vi "SendCmd.vi"(6 "HighPriority (F)":bool, 7 "UICmd":string, 8 "error in":errorcluster, 9 "Control Data":variant, 10 "Control Label":string, 11 "Queue in":refnum<queue>) -> (0 "error out":errorcluster)   [LabVIEW 2018, in "UI_Library.lvlib"]
uses:
  UI_Library.lvlib
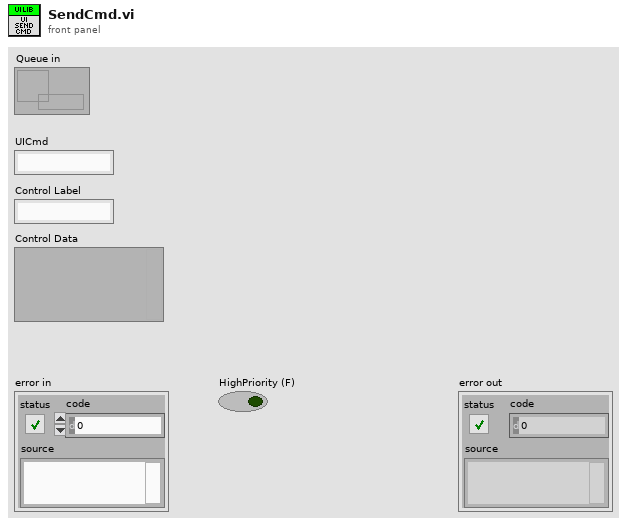
[diagram p1: front panel]
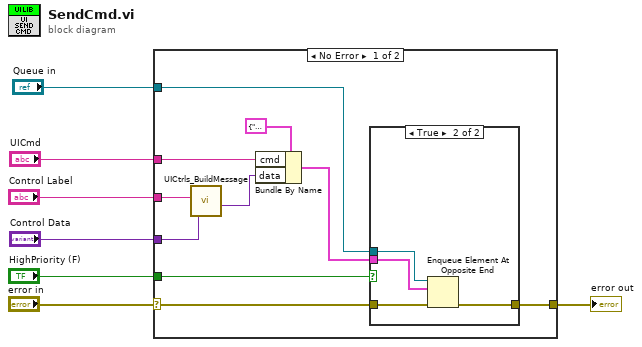
[diagram p0: block diagram]
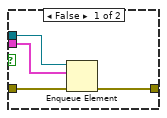
[diagram p2: hidden frame]
diagram:
  n1 = case shown="No Error" "error in" {
    selector: "error in" -> [w9 w26]
    tunnel: "Queue in" -> [w17 _]
    tunnel: "Control Label" -> [w13 _]
    tunnel: "Control Data" -> [w12 _]
    tunnel: "UICmd" -> [w11 _]
    tunnel: "HighPriority (F)" -> [w10 _]
    tunnel: [w8 w26] -> w7
    frame No Error {
      n2 = call "UICtrls_BuildMessage.vi"("Control Label"=w13, "Control Data"=w12) -> ("Data"=w14:variant)  [unwired: 6 in]
      n3 = Bundle By Name(cluster=cluster{"cmd":string, "data":variant} {"cmd"="", "data"=variant} ("element"), "cmd"=w11, "data"=w14) -> (w15:cluster{"cmd":string, "data":variant})
      n4 = case shown="True" w10 {
        tunnel: w17 -> [w21 w24]
        tunnel: w15 -> [w20 w23]
        tunnel: w9 -> [w19 w25]
        tunnel: [w18 w22] -> w8
        frame False {
          n5 = Enqueue Element(queue=w21, element=w20, error in (no error)=w19) -> (error out=w18:errorcluster)  [unwired: 1 in, 2 out]
        }
        frame True {
          n6 = Enqueue Element At Opposite End(queue=w24, element=w23, error in (no error)=w25) -> (error out=w22:errorcluster)  [unwired: 1 in, 2 out]
        }
      }
    }
    frame Error {
    }
  }
  "error out" <- w7
